vi "Calculator Example.vi"() -> ()   [LabVIEW 2012]
doc: "This VI demonstrates how to use a LabVIEW XControl. The Calculator XControl can manipulate values similar to a handheld calculator. The value of the XControl is the current calculated value shown in <b>Output</b>. \n\nOpen the Calculator XControl Project included with this example to see the configuration of the XControl."
uses:
  XControl/Calculator XControl.xctl
panel:
  in  "Calculator XControl":dbl(xcontrol)
  out "Output Value":dbl
  in  "stop":bool
  # "Run the VI to use the calculator. You can type directly into the Formula field or use the keys on the calculator keypad to enter\nvalues. \n\nClick the <=> key or press <Enter> on the keyboard to evaluate the current formula and display the solution in the Output field. You can change the digits of precision and format of the Output display using the controls at top. \n\nUse the <ans> button on the Symbol tab as a variable for the last calculated output value. Press the <CLR> button to clear the Formula field.\n\n\nSelect Help»Show Context Help and move the cursor over the VI icon to display help for this VI."
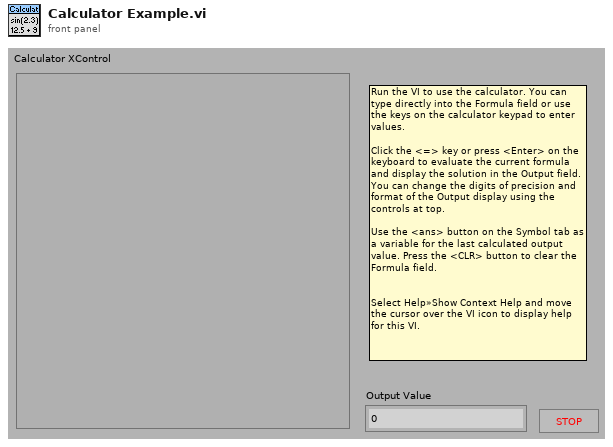
[diagram p1: front panel]
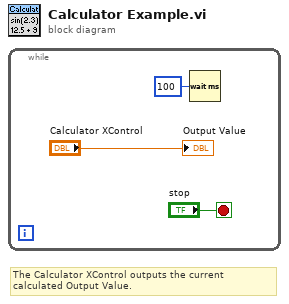
[diagram p0: block diagram]
diagram:
  # "The Calculator XControl outputs the current calculated Output Value."
  n1 = while {
    stop <- "stop" stop-if-true
    n2 = Wait (ms)(milliseconds to wait=u32 100) -> ()  [unwired: 1 out]
    "Output Value" <- "Calculator XControl"
  }
